vi "Update Snake On-Board.vi"(8 "error in (no error)":errorcluster, 11 "Game Board in":refnum<class "Game Board.lvclass">) -> (0 "error out":errorcluster, 3 "Game Board out":refnum<class "Game Board.lvclass">)   [LabVIEW 2018, in "Game Board.lvclass"]
uses:
  Game Board.lvclass
  Game Board.lvclass/Game Board.ctl
  Snake/Snake.lvclass
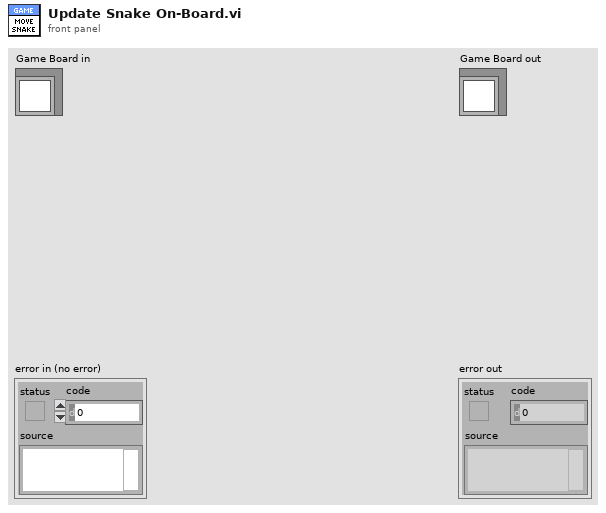
[diagram p1: front panel]
types:
  T1 = typedef "Coordinates.ctl" = cluster{"X":i32, "Y":i32}
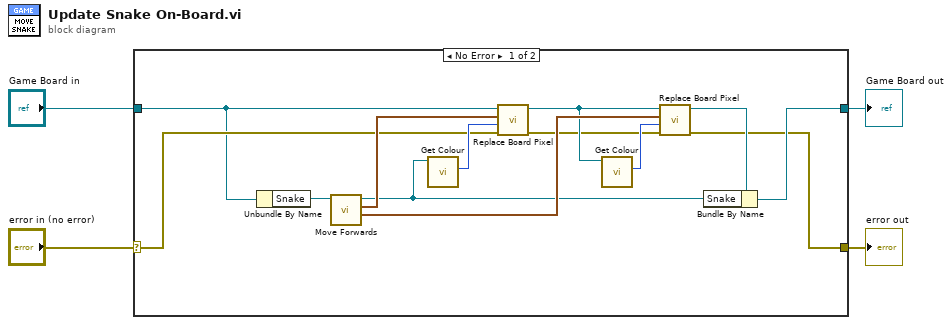
[diagram p0: block diagram]
diagram:
  n1 = case shown="No Error" "error in (no error)" {
    selector: "error in (no error)" -> [w7 w19]
    tunnel: [w9 w19] -> w3
    tunnel: [w17 w18] -> w1
    tunnel: "Game Board in" -> [w6 w18]
    frame No Error {
      n2 = Unbundle By Name(w6) -> ("Snake"=w10:refnum<class "Snake.lvclass">)
      n3 = call "Move Forwards.vi"("Snake in"=w10) -> ("Deleted Tail"=w13:T1, "New Head"=w12:T1, "Snake out"=w5:refnum<class "Snake.lvclass">)  [unwired: 7 in, 1 out]
      n4 = call-dynamic "Get Colour.vi"("Game Componants in"=w5) -> ("Componant Colour"=w16:u32)  [unwired: 10 in]
      n5 = call "Replace Board Pixel.vi"("error in (no error)"=w7, "Colour"=w16, "Coordinates"=w12, "Game Board in"=w6) -> ("error out"=w8:errorcluster, "Game Board out"=w11:refnum<class "Game Board.lvclass">)  [unwired: 6 in]
      n6 = call-dynamic "Get Colour.vi"("Game Componants in"=w11) -> ("Componant Colour"=w15:u32)  [unwired: 10 in]
      n7 = call "Replace Board Pixel.vi"("error in (no error)"=w8, "Colour"=w15, "Coordinates"=w13, "Game Board in"=w11) -> ("error out"=w9:errorcluster, "Game Board out"=w14:refnum<class "Game Board.lvclass">)  [unwired: 6 in]
      n8 = Bundle By Name(cluster=w14, "Snake"=w5) -> (w17:refnum<class "Game Board.lvclass">)
    }
    frame Error {
    }
  }
  "error out" <- w3
  "Game Board out" <- w1
